vi "sense_state.vi"(0 "state in":T1={"State"=enum."sense", "Maze"=[[FALSE, FALSE, FALSE, FALSE, FALSE, FALSE, FALSE, FALSE, FALSE], [FALSE, FALSE, TRUE, FALSE, FALSE, TRUE, TRUE, TRUE, FALSE], [FALSE, FALSE, TRUE, TRUE, TRUE, TRUE, FALSE, FALSE, FALSE], [FALSE, FALSE, TRUE, FALSE, FALSE, TRUE, FALSE, FALSE, FALSE], [TRUE, TRUE, TRUE, FALSE, FALSE, TRUE, FALSE, TRUE, TRUE], [FALSE, FALSE, FALSE, TRUE, TRUE, TRUE, FALSE, TRUE, FALSE], [FALSE, FALSE, FALSE, FALSE, FALSE, TRUE, TRUE, TRUE, FALSE], [FALSE, FALSE, FALSE, FALSE, FALSE, FALSE, FALSE, FALSE, FALSE], [FALSE, FALSE, FALSE, FALSE, FALSE, FALSE, FALSE, FALSE, FALSE]], "Runner Row"=0, "Runner Column"=0, "Runner Direction"=enum."east", "Sense"={"wall in front"=FALSE, "wall to left"=FALSE, "wall to right"=FALSE, "wall behind"=FALSE, "exit column"=FALSE}, "Hand"=enum."Left-handed"}) -> (4 "state out":T1={"State"=enum."sense", "Maze"=[[FALSE, FALSE, FALSE, FALSE, FALSE, FALSE, FALSE, FALSE, FALSE], [FALSE, FALSE, TRUE, FALSE, FALSE, TRUE, TRUE, TRUE, FALSE], [FALSE, FALSE, TRUE, TRUE, TRUE, TRUE, FALSE, FALSE, FALSE], [FALSE, FALSE, TRUE, FALSE, FALSE, TRUE, FALSE, FALSE, FALSE], [TRUE, TRUE, TRUE, FALSE, FALSE, TRUE, FALSE, TRUE, TRUE], [FALSE, FALSE, FALSE, TRUE, TRUE, TRUE, FALSE, TRUE, FALSE], [FALSE, FALSE, FALSE, FALSE, FALSE, TRUE, TRUE, TRUE, FALSE], [FALSE, FALSE, FALSE, FALSE, FALSE, FALSE, FALSE, FALSE, FALSE], [FALSE, FALSE, FALSE, FALSE, FALSE, FALSE, FALSE, FALSE, FALSE]], "Runner Row"=0, "Runner Column"=0, "Runner Direction"=enum."east", "Sense"={"wall in front"=FALSE, "wall to left"=FALSE, "wall to right"=FALSE, "wall behind"=FALSE, "exit column"=FALSE}, "Hand"=enum."Left-handed"})   [LabVIEW 2016]
uses:
  typedefs/state.ctl
  typedefs/action_start.ctl
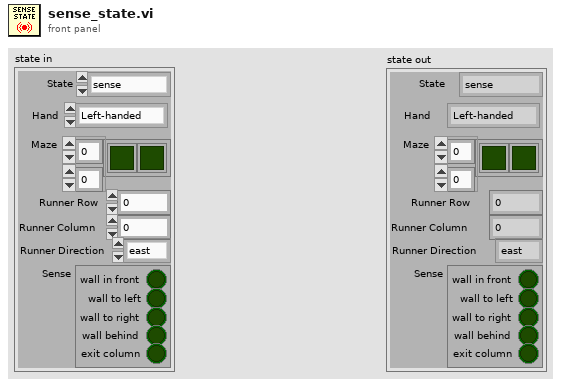
[diagram p1: front panel]
types:
  T1 = typedef "state.ctl" = cluster{"State":T2, "Maze":bool[][], "Runner Row":i32, "Runner Column":i32, "Runner Direction":enum16{"east", "north", "west", "south"}, "Sense":cluster{"wall in front":bool, "wall to left":bool, "wall to right":bool, "wall behind":bool, "exit column":bool}, "Hand":enum16{"Left-handed", "Right-handed"}}
  T2 = typedef "action_start.ctl" = enum16{"sense", "decide", "step", "pivot right", "pivot left", "stop"}
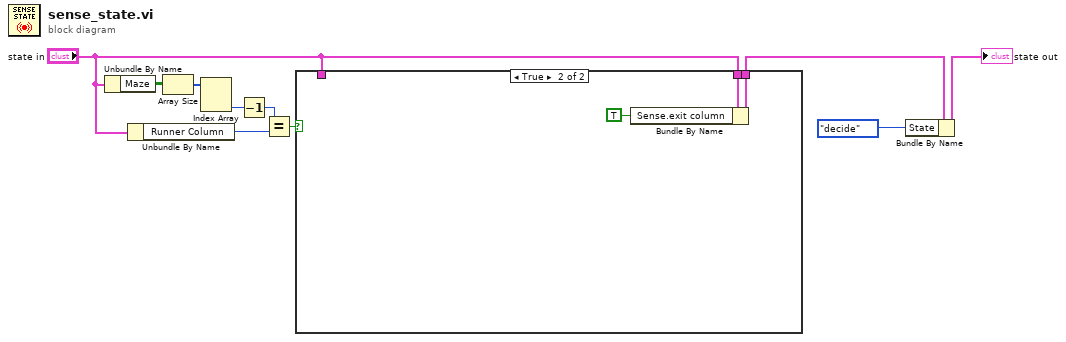
[diagram p0: block diagram]
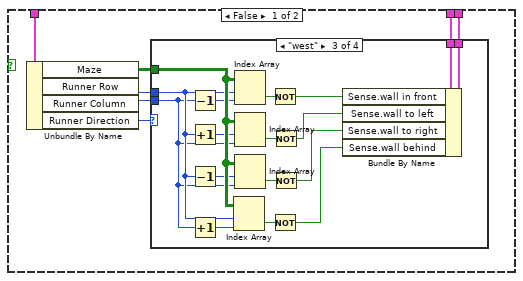
[diagram p2: hidden frame]
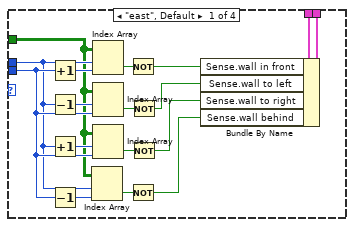
[diagram p3: hidden frame]
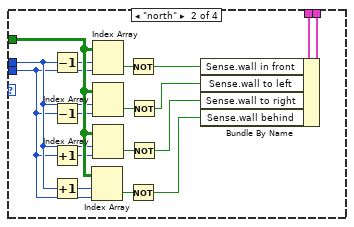
[diagram p4: hidden frame]
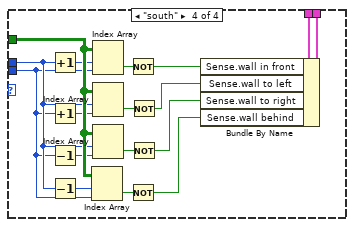
[diagram p5: hidden frame]
diagram:
  n1 = Unbundle By Name("state in") -> ("Maze"=w7:bool[][])
  n2 = Unbundle By Name("state in") -> ("Runner Column"=w3:i32)
  n3 = Array Size(array=w7) -> (size(s)=w6:i32[])
  n4 = Index Array(array=w6) -> (element #2=w4:i32)  [unwired: 2 in, 1 out]
  n5 = Decrement(x=w4) -> (x-1=w1:i32)
  n6 = Equal?(x=w1, y=w3) -> (x = y?=w2:bool)
  n7 = case shown="True" w2 {
    tunnel: "state in" -> [w13 _]
    tunnel: [w12 w87] -> w10
    tunnel: "state in" -> [w11 w88]
    frame False {
      n8 = Unbundle By Name(w13) -> ("Maze"=w15:bool[][], "Runner Row"=w17:i32, "Runner Column"=w16:i32, "Runner Direction"=w14:enum16{"east", "north", "west", "south"})
      n9 = case shown="\"west\"" w14 {
        tunnel: w17 -> [w27 w40 w57 w74]
        tunnel: w16 -> [w28 w39 w56 w73]
        tunnel: w15 -> [w24 w47 w64 w81]
        tunnel: w11 -> [w19 w42 w59 w76]
        tunnel: [w18 w41 w58 w75] -> w12
        frame "east", Default {
          n10 = Increment(x=w28) -> (x+1=w31:i32)
          n11 = Decrement(x=w27) -> (x-1=w34:i32)
          n12 = Increment(x=w27) -> (x+1=w29:i32)
          n13 = Decrement(x=w28) -> (x-1=w25:i32)
          n14 = Index Array(array=w24, index (row)=w27, index (col)=w25) -> (element=w26:bool)
          n15 = Index Array(array=w24, index (row)=w27, index (col)=w31) -> (element=w32:bool)
          n16 = Index Array(array=w24, index (row)=w34, index (col)=w28) -> (element=w33:bool)
          n17 = Index Array(array=w24, index (row)=w29, index (col)=w28) -> (element=w30:bool)
          n18 = Not(x=w32) -> (.not. x?=w23:bool)
          n19 = Not(x=w26) -> (.not. x?=w20:bool)
          n20 = Not(x=w33) -> (.not. x?=w22:bool)
          n21 = Not(x=w30) -> (.not. x?=w21:bool)
          n22 = Bundle By Name(cluster=w19, "Sense.wall in front"=w23, "Sense.wall to left"=w22, "Sense.wall to right"=w21, "Sense.wall behind"=w20) -> (w18:T1)
        }
        frame "north" {
          n23 = Decrement(x=w40) -> (x-1=w38:i32)
          n24 = Decrement(x=w39) -> (x-1=w36:i32)
          n25 = Increment(x=w39) -> (x+1=w35:i32)
          n26 = Increment(x=w40) -> (x+1=w37:i32)
          n27 = Index Array(array=w47, index (row)=w37, index (col)=w39) -> (element=w48:bool)
          n28 = Index Array(array=w47, index (row)=w38, index (col)=w39) -> (element=w50:bool)
          n29 = Index Array(array=w47, index (row)=w40, index (col)=w36) -> (element=w51:bool)
          n30 = Index Array(array=w47, index (row)=w40, index (col)=w35) -> (element=w49:bool)
          n31 = Not(x=w50) -> (.not. x?=w46:bool)
          n32 = Not(x=w48) -> (.not. x?=w43:bool)
          n33 = Not(x=w51) -> (.not. x?=w45:bool)
          n34 = Not(x=w49) -> (.not. x?=w44:bool)
          n35 = Bundle By Name(cluster=w42, "Sense.wall in front"=w46, "Sense.wall to left"=w45, "Sense.wall to right"=w44, "Sense.wall behind"=w43) -> (w41:T1)
        }
        frame "west" {
          n36 = Decrement(x=w56) -> (x-1=w55:i32)
          n37 = Increment(x=w57) -> (x+1=w53:i32)
          n38 = Decrement(x=w57) -> (x-1=w52:i32)
          n39 = Increment(x=w56) -> (x+1=w54:i32)
          n40 = Index Array(array=w64, index (row)=w57, index (col)=w54) -> (element=w65:bool)
          n41 = Index Array(array=w64, index (row)=w57, index (col)=w55) -> (element=w67:bool)
          n42 = Index Array(array=w64, index (row)=w53, index (col)=w56) -> (element=w68:bool)
          n43 = Index Array(array=w64, index (row)=w52, index (col)=w56) -> (element=w66:bool)
          n44 = Not(x=w67) -> (.not. x?=w63:bool)
          n45 = Not(x=w65) -> (.not. x?=w60:bool)
          n46 = Not(x=w68) -> (.not. x?=w62:bool)
          n47 = Not(x=w66) -> (.not. x?=w61:bool)
          n48 = Bundle By Name(cluster=w59, "Sense.wall in front"=w63, "Sense.wall to left"=w62, "Sense.wall to right"=w61, "Sense.wall behind"=w60) -> (w58:T1)
        }
        frame "south" {
          n49 = Increment(x=w74) -> (x+1=w72:i32)
          n50 = Increment(x=w73) -> (x+1=w70:i32)
          n51 = Decrement(x=w73) -> (x-1=w69:i32)
          n52 = Decrement(x=w74) -> (x-1=w71:i32)
          n53 = Index Array(array=w81, index (row)=w71, index (col)=w73) -> (element=w82:bool)
          n54 = Index Array(array=w81, index (row)=w72, index (col)=w73) -> (element=w84:bool)
          n55 = Index Array(array=w81, index (row)=w74, index (col)=w70) -> (element=w85:bool)
          n56 = Index Array(array=w81, index (row)=w74, index (col)=w69) -> (element=w83:bool)
          n57 = Not(x=w84) -> (.not. x?=w80:bool)
          n58 = Not(x=w82) -> (.not. x?=w77:bool)
          n59 = Not(x=w85) -> (.not. x?=w79:bool)
          n60 = Not(x=w83) -> (.not. x?=w78:bool)
          n61 = Bundle By Name(cluster=w76, "Sense.wall in front"=w80, "Sense.wall to left"=w79, "Sense.wall to right"=w78, "Sense.wall behind"=w77) -> (w75:T1)
        }
      }
    }
    frame True {
      n62 = Bundle By Name(cluster=w88, "Sense.exit column"=TRUE ("sense.exit column")) -> (w87:T1)
    }
  }
  n63 = Bundle By Name(cluster=w10, "State"=action_start."decide" ("action")) -> (→"state out":T1)
